vi "基于延迟的串口通信组件(Slave).vi"(5 "error in":errorcluster) -> (11 "Stop":bool, 19 "error out":errorcluster)   [LabVIEW 2013]
uses:
  <vilib>/Instr/_visa.llb/VISA Configure Serial Port (Instr).vi
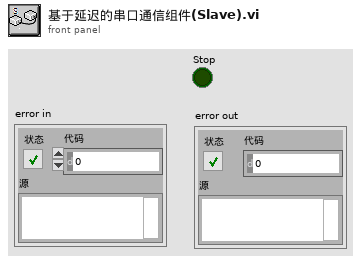
[diagram p1: front panel]
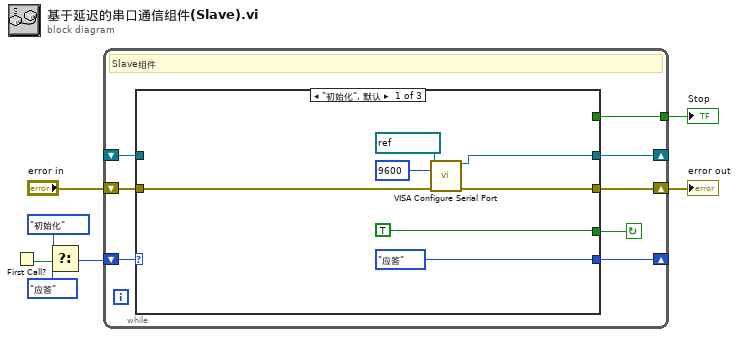
[diagram p0: block diagram]
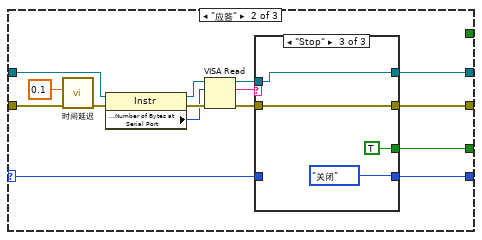
[diagram p2: hidden frame]
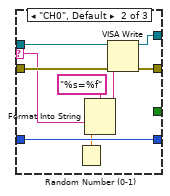
[diagram p4: hidden frame]
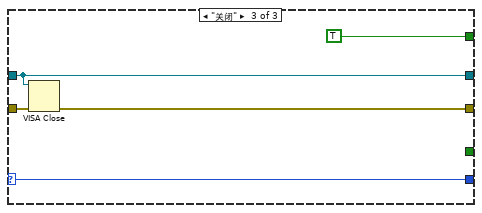
[diagram p5: hidden frame]
diagram:
  n1 = First Call?() -> (First Call?: T/F=w7:bool)
  n2 = Select(t=enum16{"初始化", "应答", "关闭"}."初始化" ("枚举"), s=w7, f=enum16{"初始化", "应答", "关闭"}."应答" ("枚举")) -> (s? t:f=w6:enum16{"初始化", "应答", "关闭"})
  n3 = while {
    shift-right: [w15] -> w3
    shift-left: "error in" -> [w13]
    shift-right: [w14] -> _
    shift-left: _ -> [w12]
    shift-right: [w11] -> _
    shift-left: w6 -> [w10]
    tunnel: [w8] -> w1
    stop <- w9 continue-if-true
    # "Slave组件"
    n4 = case shown="\"初始化\", 默认" w10 {
      selector: w10 -> [_ w26 w55]
      tunnel: [w20 w25 w56] -> w14
      tunnel: [w19 w24 w57] -> w15
      tunnel: w13 -> [w18 w29 w58]
      tunnel: w12 -> [_ w28 w56]
      tunnel: [TRUE w30 _] -> w9
      tunnel: [enum16{"初始化", "应答", "关闭"}."应答" ("枚举") w27 w55] -> w11
      tunnel: [_ _ TRUE] -> w8
      frame "初始化", Default {
        n5 = call-poly "VISA Configure Serial Port"("VISA resource name"=refnum<visa-resource-name> "COM3", "baud rate (9600)"=u32 9600, "error in (no error)"=w18) -> ("VISA resource name out"=w20:refnum<visa-resource-name>, "error out"=w19:errorcluster)  [unwired: 11 in]
      }
      frame "应答" {
        n6 = call "时间延迟"("error in (no error)"=w29, "Delay Time (s)"=0.1) -> ("error out"=w32:errorcluster)  [unwired: 9 in]
        n7 = property class="Instr"(reference=w28, error in=w32) -> (reference out=w33:refnum<visa-resource-name>, error out=w35:errorcluster, "Serial Settings:Number of Bytes at Serial Port"=w34:u32)
        n8 = VISA Read(VISA resource name=w33, byte count=w34, error in (no error)=w35) -> (VISA resource name out=w36:refnum<visa-resource-name>, read buffer=w23:string, error out=w37:errorcluster)  [unwired: 1 out]
        n9 = case shown="\"Stop\"" w23 {
          selector: w23 -> [_ w42 _]
          tunnel: w36 -> [w39 w48 w53]
          tunnel: [w39 w47 w53] -> w25
          tunnel: w37 -> [w38 w49 w52]
          tunnel: [w38 w46 w52] -> w24
          tunnel: [_ _ TRUE] -> w30
          tunnel: [w40 w45 enum16{"初始化", "应答", "关闭"}."关闭" ("枚举")] -> w27
          tunnel: w26 -> [w40 w45 _]
          frame "" {
          }
          frame "CH0", Default {
            n10 = Random Number (0-1)() -> (number: 0 to 1=w43:dbl)
            n11 = Format Into String(format string="%s=%f" ("格式字符串"), w42, w43) -> (resulting string=w41:string)  [unwired: 2 in, 1 out]
            n12 = VISA Write(VISA resource name=w48, write buffer=w41, error in (no error)=w49) -> (VISA resource name out=w47:refnum<visa-resource-name>, error out=w46:errorcluster)  [unwired: 1 out]
          }
          frame "Stop" {
          }
        }
      }
      frame "关闭" {
        n13 = VISA Close(VISA resource name=w56, error in (no error)=w58) -> (error out=w57:errorcluster)
      }
    }
  }
  "error out" <- w3
  "Stop" <- w1
